vi "JSON_to_StringArray.vi"(11 "body":string) -> (3 "Array":string[](array[string]))   [LabVIEW 2015]
uses:
  <vilib>/regexp/Match Regular Expression.xnode
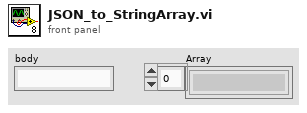
[diagram p1: front panel]
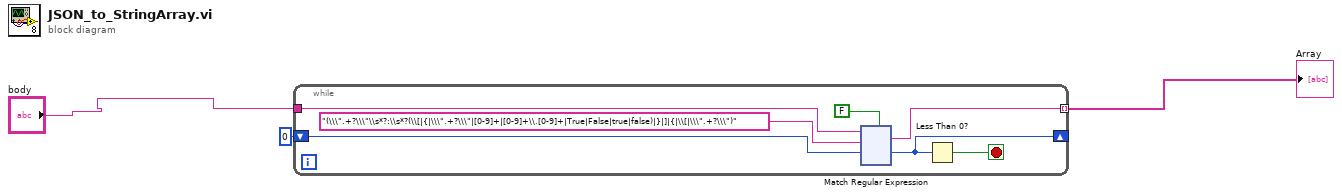
[diagram p0: block diagram]
diagram:
  n1 = while {
    tunnel: "body" -> [w9]
    shift-right: [w4] -> _
    shift-left: 0 ("offset past match") -> [w7]
    tunnel: [w6] -> w3 mode=indexing
    stop <- w10 stop-if-true
    n2 = xnode "Match Regular Expression"("input string"=w9, "regular expression"="(\\\".+?\\\"\\s*?:\\s*?(\\[|{|\\\".+?\\\"|[0-9]+|[0-9]+\\.[0-9]+|True|False|true|false)|}|]|{|\\[|\\\".+?\\\")", "offset (0)"=w7, "multiline? (F)"=FALSE) -> ("whole match"=w6:string, "offset past match"=w4:i32)  [unwired: 2 in, 3 out]
    n3 = Less Than 0?(x=w4) -> (x < 0?=w10:bool)
  }
  "Array" <- w3
